vi "HOST.vi"() -> ()   [LabVIEW 2017]
uses:
  <vilib>/Platform/TimedLoop/XDataNode/timing_clust.ctl
  <vilib>/Platform/TimedLoop/XDataNode/nitl_modes.ctl
  <vilib>/Platform/TimedLoop/XDataNode/wakeup.ctl
  <vilib>/Platform/TimedLoop/XDataNode/XDataNode.xnode
  <vilib>/Platform/TimedLoop/XDataNode/XDNodeRunTimeDep.lvlib
panel:
  out "Consumed air":dbl
  out "ECO mode":bool
  out "Log file directory":path
  in  "Choose folder":bool
  in  "Enable":bool=TRUE
  out "Saving Data":bool
  out "Meter":dbl(knob) scale=0.0..80.0
  in  "stop":bool
  out "Gauge":dbl(knob) scale=0.0..2000.0
  in  "Clear charts":bool
  in  "Basic control":refnum<k24>(container)
  out "Horizontal Progress Bar":u8(slide) scale=0.0..100.0
  in  "Filename":path=path "C:/Users/Student/Desktop/Pneumobil/Laboratorium/test.lvm"
  out "Vehicle - piston velocity diagram":cluster{"X":dbl[], "Y":dbl[]}[](graph)
  out "Velocity of the vehicle":dbl(graph)
  out "Displacement - force diagram":cluster{"X":dbl[], "Y":dbl[]}[](graph)
  out "Piston position":dbl(graph)
  out "Air consumption":dbl(graph)
  in  "reset":bool
  # "liters"
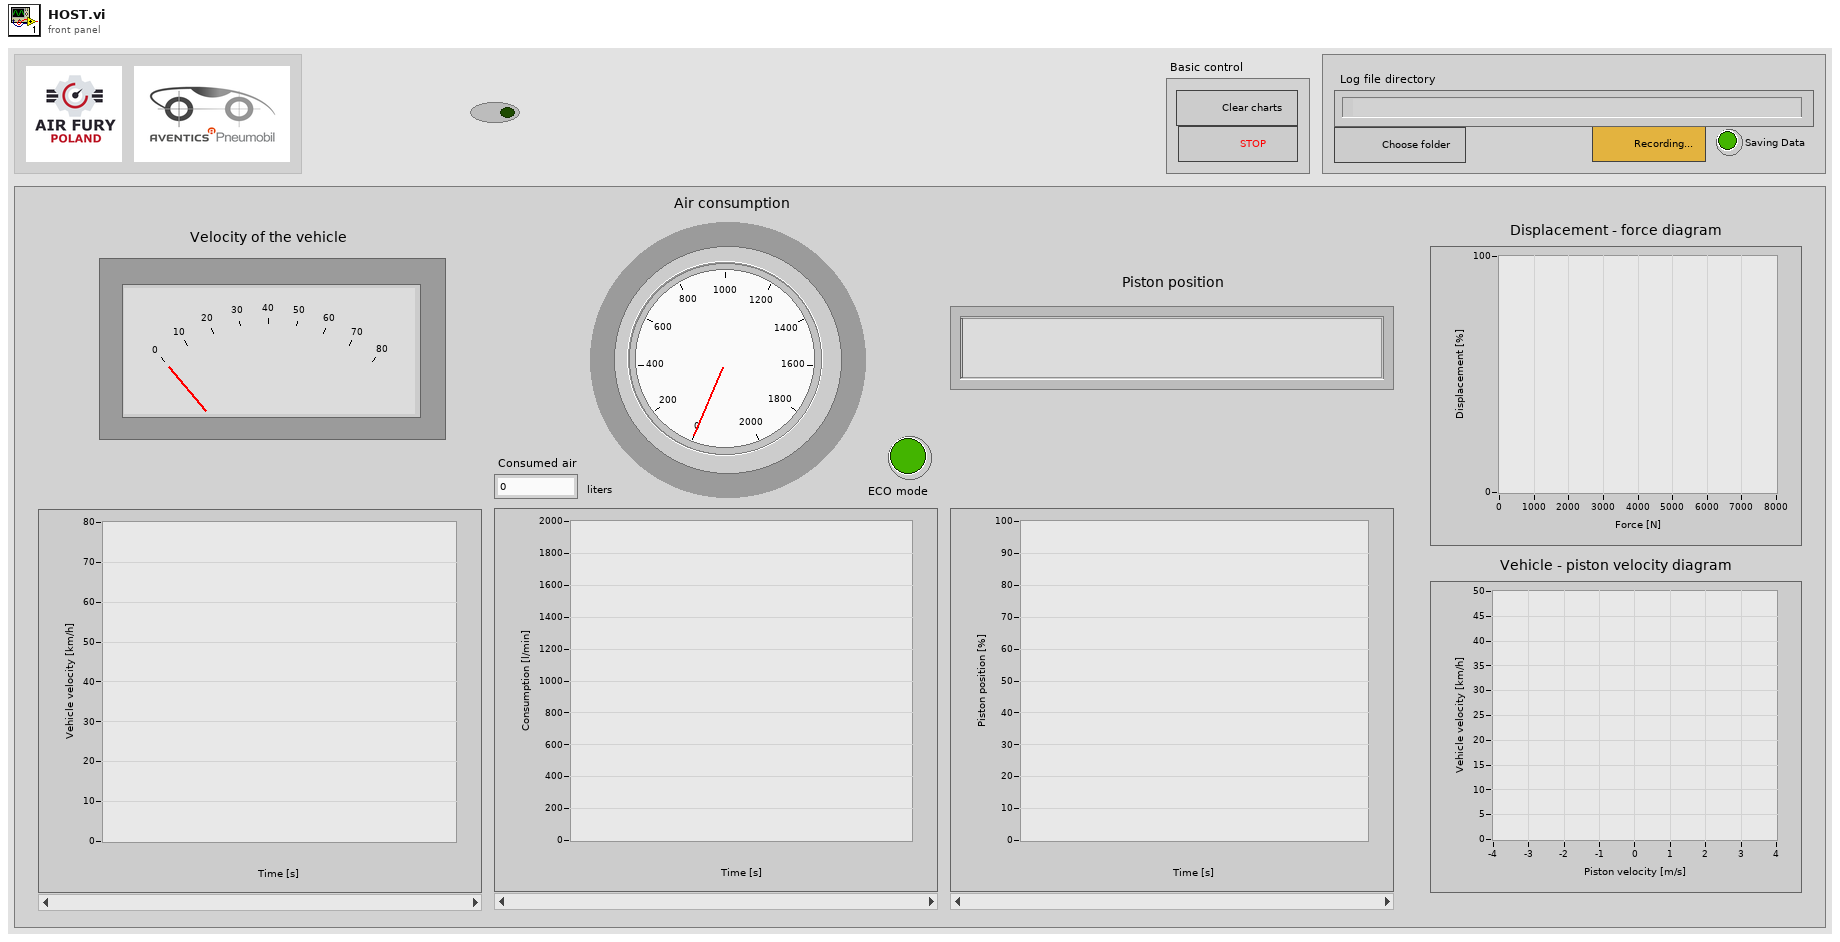
[diagram p1: front panel]
types:
  T1 = typedef "XDNodeRunTimeDep.lvlib/timing_clust.ctl" = cluster{"Expected End [f-1]":u64, "Actual End [f-1]":u64, "Finished Late? [f-1]":bool, "Expected End [i-1]":u64, "Actual End [i-1]":u64, "Finished Late? [i-1]":bool, "Expected Start [i]":u64, "Actual Start [i]":u64, "Expected Start [f]":u64, "Actual Start [f]":u64, "Source Name":string, "Structure Name":string, "Period":i64, "Deadline":i64, "Offset":i64, "Start":i64, "Priority":i32, "Timeout":i32, "Mode":T2, "Wakeup Reason":T3, "Error":errorcluster, "Source Type":string, "Secondary Source Type":string, "Global End Time":u64, "Global Start Time":u64, "Frame Duration":u64, "Iteration Duration":u64, "Assigned CPU":i32, "I/O Scan Engine Mode":u32}
  T2 = typedef "XDNodeRunTimeDep.lvlib/nitl_modes.ctl" = enum32{"No Change", "Process missed periods, maintain original phase", "Discard missed periods, maintain original phase", "Process missed periods, ignore original phase", "Discard missed periods, ignore original phase"}
  T3 = typedef "XDNodeRunTimeDep.lvlib/wakeup.ctl" = enum32{"Normal", "Aborted", "Asynchronous wakeup", "Timing source error", "Timed loop error", "Timeout"}
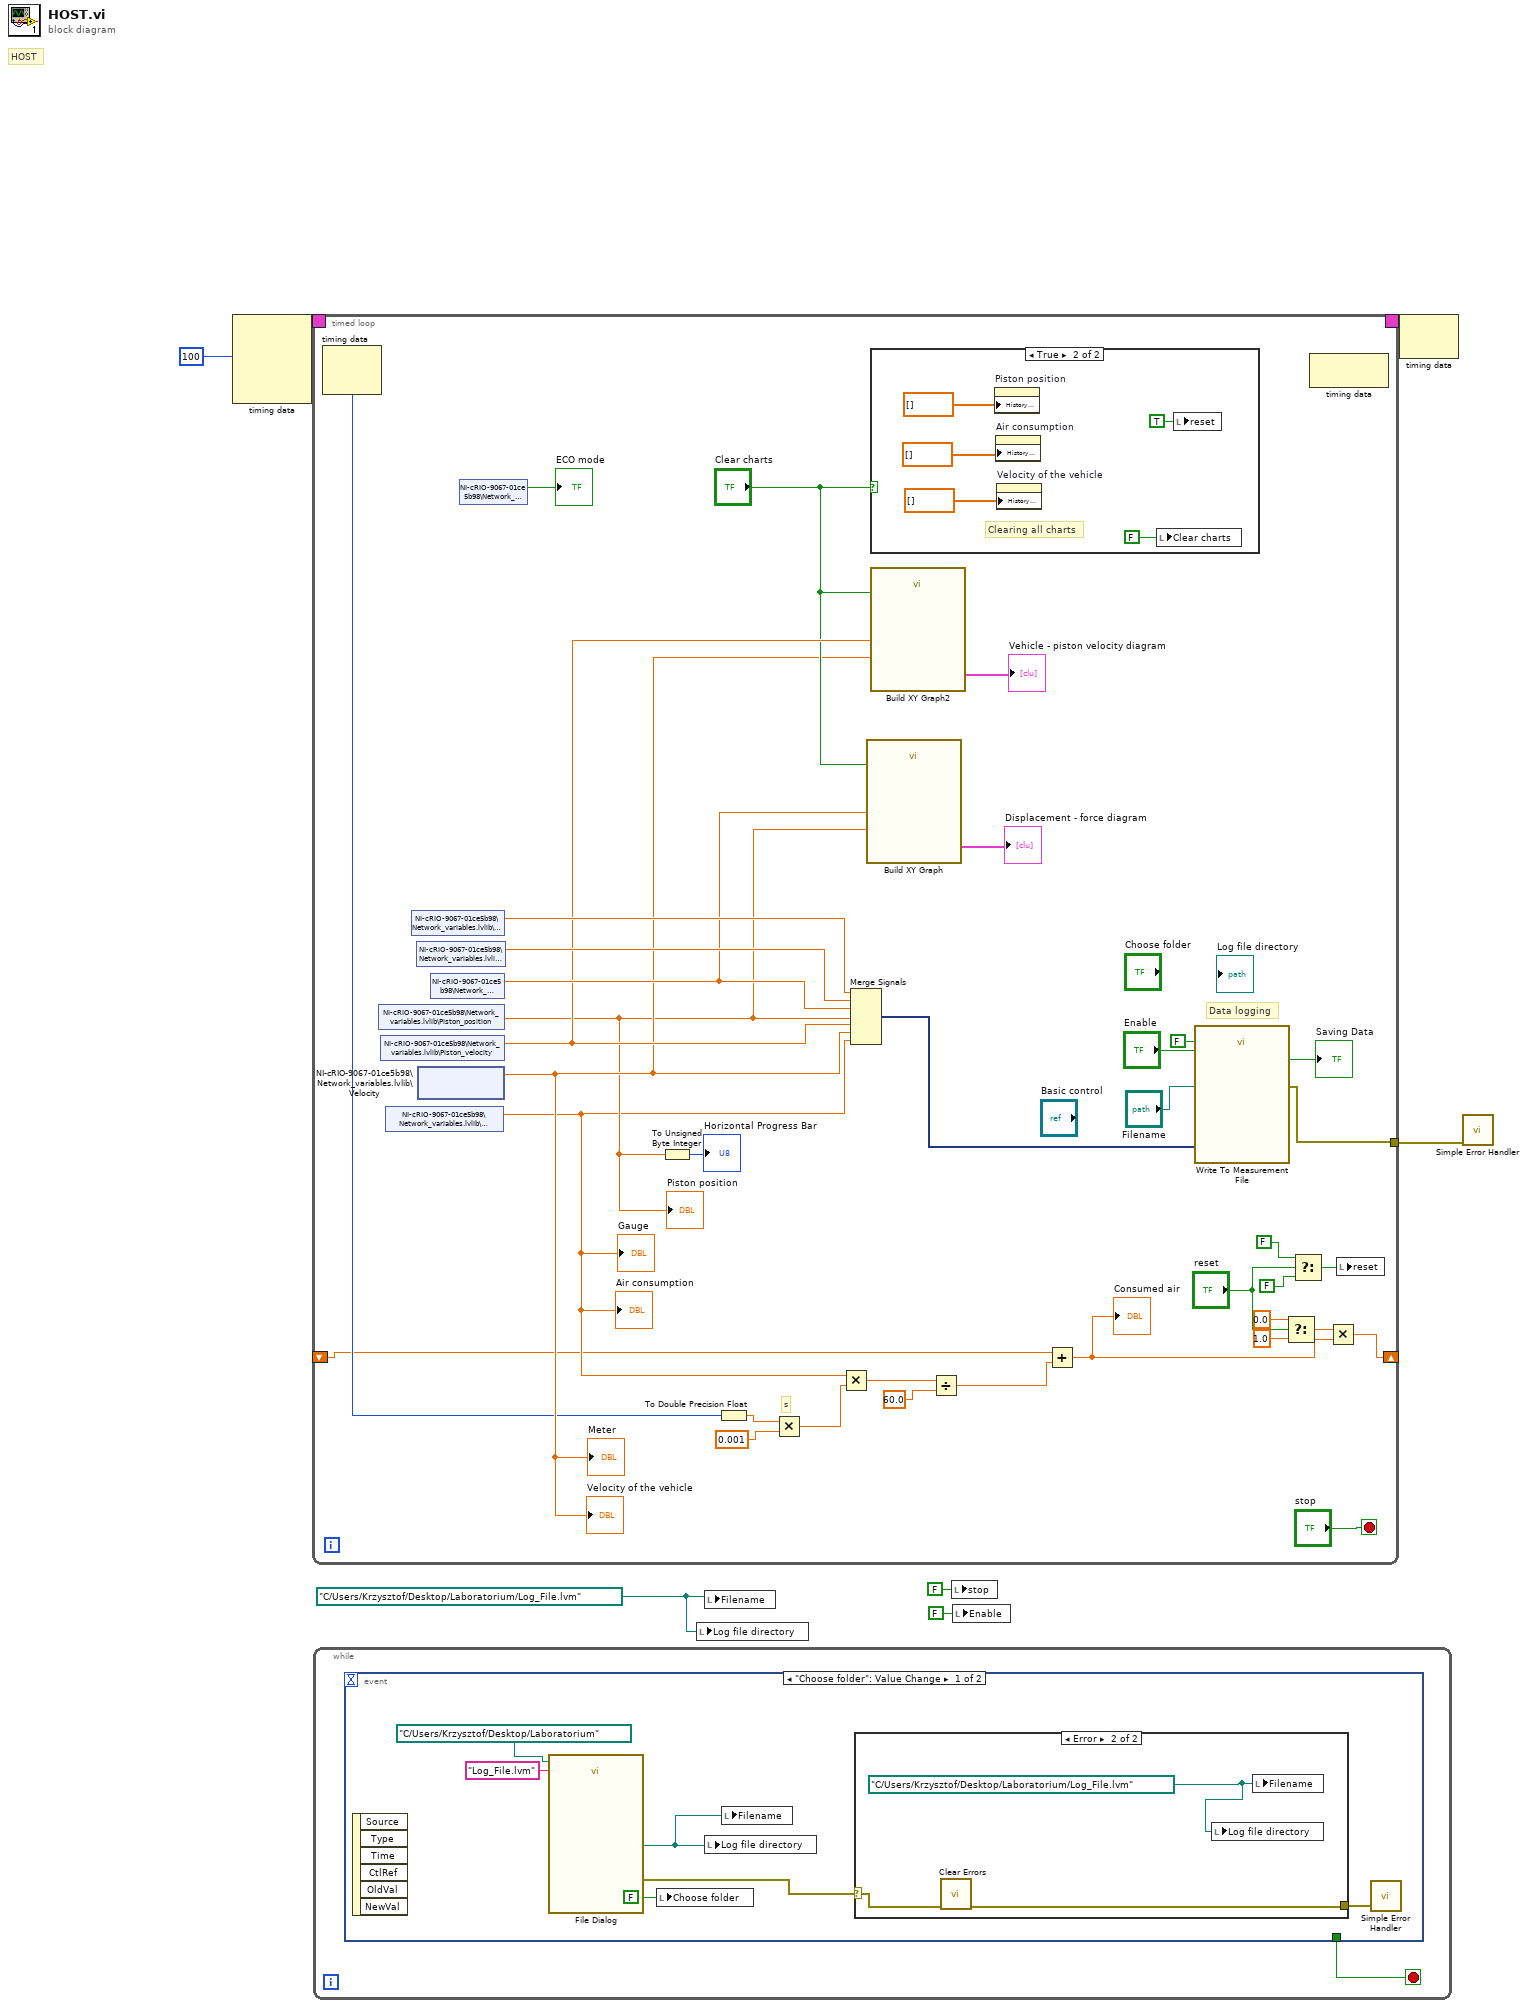
[diagram p0: block diagram]
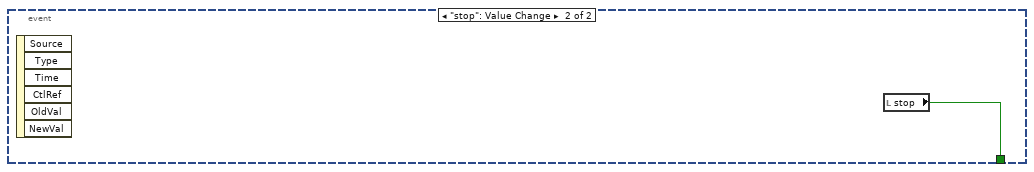
[diagram p3: hidden frame]
diagram:
  w3 = path "C:/Users/Krzysztof/Desktop/Laboratorium/Log_File.lvm"
  # "HOST"
  n1 = node-c288(i64 100 ("Period")) -> (w7:T1)  [unwired: 3 in]
  n2 = timed-loop {
    timing: w7 -> [_]
    timing-out: [_] -> w6
    tunnel: [w41] -> w4
    shift-right: [w8] -> _
    shift-left: _ -> [w20]
    stop <- "stop" stop-if-true
    # "s"
    # "Data logging"
    n3 = node-c288() -> (w23:i64)  [unwired: 1 in, 1 out]
    n4 = shared-variable "NI-cRIO-9067-01ce5b98\\Network_variables.lvlib\\Piston_position"() -> (w27:dbl)  [unwired: 1 in, 1 out]
    "Piston position" <- w27
    n5 = shared-variable "NI-cRIO-9067-01ce5b98\\Network_variables.lvlib\\Piston_velocity"() -> (w35:dbl)  [unwired: 1 in, 1 out]
    n6 = shared-variable "NI-cRIO-9067-01ce5b98\\Network_variables.lvlib\\Consumption"() -> (w22:dbl)  [unwired: 1 in, 1 out]
    "Air consumption" <- w22
    "Gauge" <- w22
    n7 = shared-variable "NI-cRIO-9067-01ce5b98\\Network_variables.lvlib\\Pedal_tilt"() -> (w39:dbl)  [unwired: 1 in, 1 out]
    n8 = shared-variable "NI-cRIO-9067-01ce5b98\\Network_variables.lvlib\\Pressure"() -> (w42:dbl)  [unwired: 1 in, 1 out]
    n9 = shared-variable "NI-cRIO-9067-01ce5b98\\Network_variables.lvlib\\Velocity"() -> (w28:dbl)  [unwired: 1 in, 2 out]
    "Velocity of the vehicle" <- w28
    "Meter" <- w28
    n10 = shared-variable "NI-cRIO-9067-01ce5b98\\Network_variables.lvlib\\Force"() -> (w36:dbl)  [unwired: 1 in, 1 out]
    n11 = shared-variable "NI-cRIO-9067-01ce5b98\\Network_variables.lvlib\\ECO"() -> (→"ECO mode":bool)  [unwired: 1 in, 1 out]
    n12 = To Unsigned Byte Integer(number=w27) -> (unsigned 8bit integer=→"Horizontal Progress Bar":u8)
    n13 = To Double Precision Float(number=w23) -> (double precision float=w25:dbl)
    n14 = Multiply(x=w25, y=0.001 ("x")) -> (x*y=w21:dbl)
    n15 = Multiply(x=w22, y=w21) -> (x*y=w19:dbl)
    n16 = Merge Signals(w39, w42, w36, w27, w35, w28, w22) -> (w30:dynamicdata)
    n17 = call "Build XY Graph"("Reset"="Clear charts", "Y Input"=w27, "X Input"=w36) -> ("XY Graph"=→"Displacement - force diagram":cluster{"X":dbl[], "Y":dbl[]}[])  [unwired: 7 in, 1 out]
    n18 = case shown="True" "Clear charts" {
      frame False {
      }
      frame True {
        # "Clearing all charts"
        n19 = property on="Piston position" class="WFChart (strict)"("History Data"=dbl[] []) -> ()  [unwired: 2 in, 2 out]
        n20 = property on="Air consumption" class="WFChart (strict)"("History Data"=dbl[] []) -> ()  [unwired: 2 in, 2 out]
        n21 = property on="Velocity of the vehicle" class="WFChart (strict)"("History Data"=dbl[] []) -> ()  [unwired: 2 in, 2 out]
        n22 = local write "Clear charts"(FALSE ("Restart")) -> ()
        n23 = local write "reset"(TRUE ("reset")) -> ()
      }
    }
    n24 = call "Build XY Graph2"("Reset"="Clear charts", "Y Input"=w28, "X Input"=w35) -> ("XY Graph"=→"Vehicle - piston velocity diagram":cluster{"X":dbl[], "Y":dbl[]}[])  [unwired: 7 in, 1 out]
    n25 = Divide(x=w19, y=60.0) -> (x/y=w18:dbl)
    n26 = Add(x=w20, y=w18) -> (x+y=w9:dbl)
    "Consumed air" <- w9
    n27 = call "Write To Measurement File"("Signals"=w30, "Reset"=FALSE, "Enable"="Enable", "Filename"="Filename") -> ("Saving Data"=→"Saving Data":bool, "error out"=w41:errorcluster)  [unwired: 13 in, 1 out]
    n28 = Select(t=0.0, s="reset", f=1.0) -> (s? t:f=w10:dbl)
    n29 = Select(t=FALSE, s="reset", f=FALSE) -> (s? t:f=w13:bool)
    n30 = node-c288() -> ()  [unwired: 1 in, 1 out]
    n31 = Multiply(x=w10, y=w9) -> (x*y=w8:dbl)
    n32 = local write "reset"(w13) -> ()
  }
  n33 = while {
    stop <- w52 stop-if-true
    n34 = event shown="[0] \"Choose folder\": Value Change" {
      selector: _ -> [_ _]
      dyn-events: _ -> [_ _]
      timeout: _ -> [_ _]
      tunnel: [_ w62] -> w52
      event "Choose folder": Value Change {
        n35 = event-data() -> ()  [unwired: 1 in, 6 out]
        n36 = call "File Dialog"("start path"=path "C:/Users/Krzysztof/Desktop/Laboratorium", "default name"="Log_File.lvm") -> ("selected path"=w55:path, "error out"=w54:errorcluster)  [unwired: 10 in, 2 out]
        n37 = local write "Choose folder"(FALSE ("Choose folder")) -> ()
        n38 = local write "Log file directory"(w55) -> ()
        n39 = local write "Filename"(w55) -> ()
        n40 = case shown="Error" w54 {
          selector: w54 -> [_ w61]
          tunnel: [_ w60] -> w53
          frame No Error {
          }
          frame Error {
            w59 = path "C:/Users/Krzysztof/Desktop/Laboratorium/Log_File.lvm"
            n41 = call <vilib>:"Clear Errors.vi"("error in (no error)"=w61) -> ("error out"=w60:errorcluster)  [unwired: 5 in, 1 out]
            n42 = local write "Log file directory"(w59) -> ()
            n43 = local write "Filename"(w59) -> ()
          }
        }
        n44 = call <vilib>:"Simple Error Handler.vi"("error in (no error)"=w53) -> ()  [unwired: 4 in, 5 out]
      }
      event "stop": Value Change {
        n45 = event-data() -> ()  [unwired: 1 in, 6 out]
        n46 = local read "stop"() -> (w62:bool)
      }
    }
  }
  n47 = local write "Log file directory"(w3) -> ()
  n48 = local write "Filename"(w3) -> ()
  n49 = local write "stop"(FALSE ("stop")) -> ()
  n50 = local write "Enable"(FALSE ("Enable")) -> ()
  n51 = node-c288(w6) -> ()  [unwired: 1 out]
  n52 = call <vilib>:"Simple Error Handler.vi"("error in (no error)"=w4) -> ()  [unwired: 4 in, 5 out]
